vi "Init Game.vi"(8 "error in (no error)":errorcluster, 11 "SB App in":refnum<class "SB App.lvclass">) -> (0 "error out":errorcluster, 3 "SB App out":refnum<class "SB App.lvclass">)   [LabVIEW 2020, in "SB App.lvlib" / "SB App.lvclass"]
uses:
  SB App.lvclass
  SB App.lvclass/SB App.ctl
  SquareBattle/Game/Game.lvclass
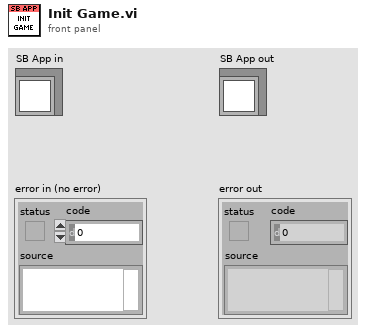
[diagram p1: front panel]
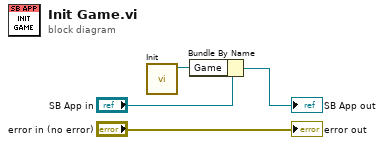
[diagram p0: block diagram]
diagram:
  n1 = call "Init.vi"() -> ("Game out"=w3:refnum<class "Game.lvclass">)  [unwired: 10 in, 1 out]
  n2 = Bundle By Name(cluster="SB App in", "Game"=w3) -> (→"SB App out":refnum<class "SB App.lvclass">)
  "error out" <- "error in (no error)"
